vi "Add file to project.vi"(8 "error in":errorcluster, 9 "Project Ref in":refnum<vi>, 11 "File Path":path[](array[path])) -> (0 "error out":errorcluster, 1 "Project out":refnum<vi>, 3 "Actual File Path":path[](array[path]))   [LabVIEW 2018]
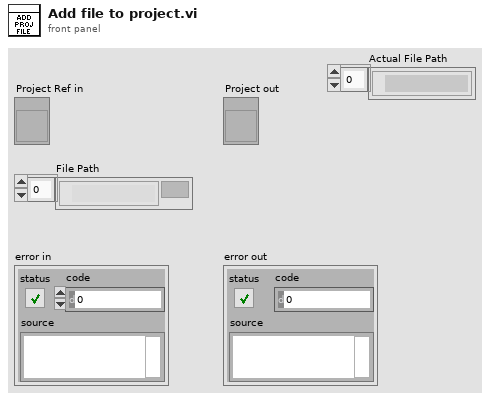
[diagram p1: front panel]
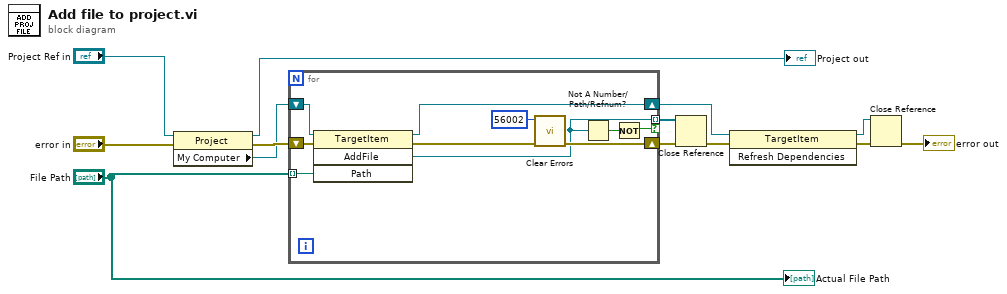
[diagram p0: block diagram]
diagram:
  n1 = property class="Project"(reference="Project Ref in", error in="error in") -> (reference out=→"Project out":refnum<vi>, error out=w9:errorcluster, "My Computer"=w8:refnum<vi>)
  n2 = for {
    tunnel: "File Path" -> [w21] mode=indexing
    shift-right: [w19] -> w2
    shift-left: w8 -> [w23]
    shift-right: [w18] -> w7
    shift-left: w9 -> [w22]
    tunnel: [w16] -> w6 mode=indexing if=w14
    n3 = invoke class="TargetItem" method="AddFile"(reference=w23, error in=w22, "Path"=w21) -> (reference out=w19:refnum<vi>, error out=w20:errorcluster, "AddFile"=w16:refnum<vi>)  [unwired: 1 in, 1 out]
    n4 = call <vilib>:"Clear Errors.vi"("error in (no error)"=w20, "specific error code to clear (0: all)"=56002) -> ("error out"=w18:errorcluster)  [unwired: 4 in, 1 out]
    n5 = Not A Number/Path/Refnum?(number/path/refnum=w16) -> (NaN/Path/Refnum?=w15:bool)
    n6 = Not(x=w15) -> (.not. x?=w14:bool)
  }
  n7 = Close Reference(reference=w6, error in (no error)=w7) -> (error out=w5:errorcluster)
  n8 = invoke class="TargetItem" method="Refresh Dependencies"(reference=w2, error in=w5) -> (reference out=w1:refnum<vi>, error out=w3:errorcluster)  [unwired: 1 in, 1 out]
  n9 = Close Reference(reference=w1, error in (no error)=w3) -> (error out=→"error out":errorcluster)
  "Actual File Path" <- "File Path"
